vi "Configure Memory Polynomial.vi"(0 "Instrument Handle In":refnum<k21>, 1 "Selector String":string, 5 "Memory Polynomial Configuration":T1={"Correction Type"=0, "Number of Iterations"=3, " Order"=3, " Depth"=2, "Lead Order"=2, "Lag Order"=2, "Lead Memory Depth"=2, "Lag Memory Depth"=2, "Maximum Lead"=2, "Maximum Lag"=2} {"Order" min=1; "Correction Type" items=["Magnitude and Phase", "Magnitude Only", "Phase Only"]}, 11 "error in (no error)":errorcluster) -> (4 "Instrument Handle Out":refnum<k21>, 15 "error out":errorcluster)   [LabVIEW 2016, in "RFmxDPD.lvlib"]
uses:
  RFmxDPD.lvlib
  Typedefs/Memory Polynomial Configuration.ctl
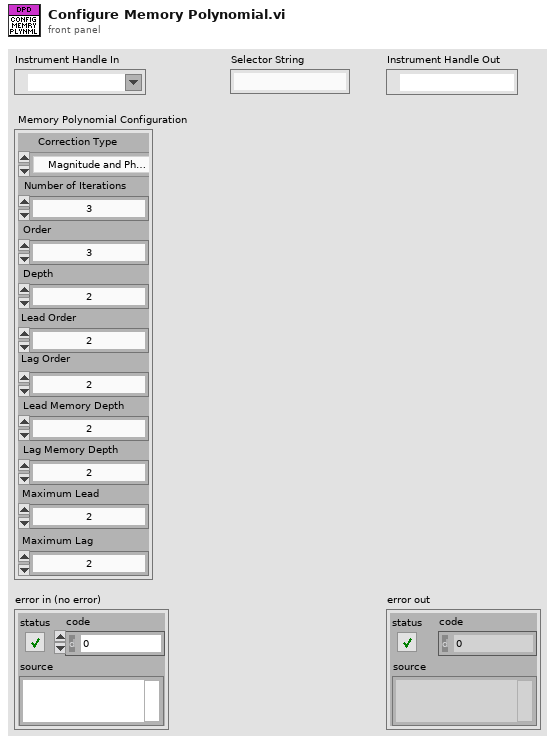
[diagram p1: front panel]
types:
  T1 = typedef "RFmxDPD.lvlib/Memory Polynomial Configuration.ctl" = cluster{"Correction Type":i32, "Number of Iterations":i32, " Order":i32, " Depth":i32, "Lead Order":i32, "Lag Order":i32, "Lead Memory Depth":i32, "Lag Memory Depth":i32, "Maximum Lead":i32, "Maximum Lag":i32}
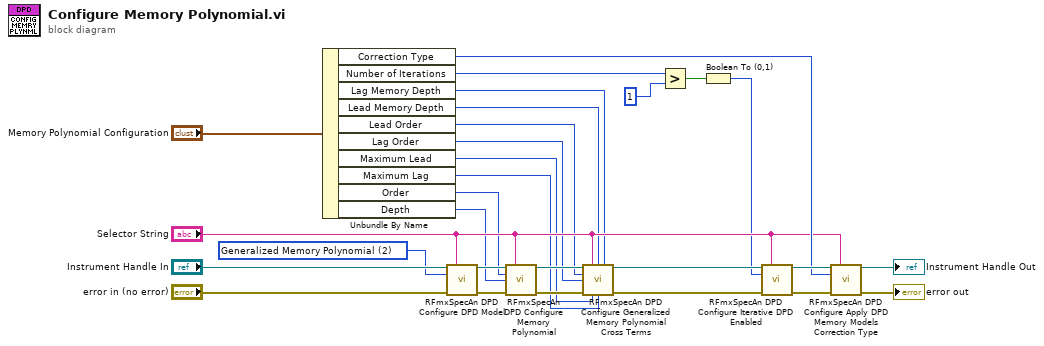
[diagram p0: block diagram]
diagram:
  w18 = 2 items=["Lookup Table", "Memory Polynomial", "Generalized Memory Polynomial"] ("DPD Model")
  n1 = Unbundle By Name("Memory Polynomial Configuration") -> ("Correction Type"=w17:i32, "Number of Iterations"=w4:i32, "Lag Memory Depth"=w15:i32, "Lead Memory Depth"=w14:i32, "Lead Order"=w13:i32, "Lag Order"=w12:i32, "Maximum Lead"=w11:i32, "Maximum Lag"=w10:i32, "Order"=w9:i32, "Depth"=w8:i32)
  n2 = call <vilib>:"RFmxSpecAn DPD Configure DPD Model.vi"("Instrument Handle In"="Instrument Handle In", "Selector String"="Selector String", "DPD Model"=w18, "error in (no error)"="error in (no error)") -> ("Instrument Handle Out"=w25:refnum<k21>, "error out"=w26:errorcluster)  [unwired: 10 in]
  n3 = call <vilib>:"RFmxSpecAn DPD Configure Memory Polynomial.vi"("Instrument Handle In"=w25, "Selector String"="Selector String", "Memory Polynomial Order"=w9, "Memory Polynomial Memory Depth"=w8, "error in (no error)"=w26) -> ("Instrument Handle Out"=w28:refnum<k21>, "error out"=w27:errorcluster)  [unwired: 9 in]
  n4 = call <vilib>:"RFmxSpecAn DPD Configure Generalized Memory Polynomial Cross Terms.vi"("Instrument Handle In"=w28, "Selector String"="Selector String", "Memory Polynomial Lead Memory Depth"=w14, "Memory Polynomial Lag Memory Depth"=w15, "Memory Polynomial Lead Order"=w13, "Memory Polynomial Lag Order"=w12, "error in (no error)"=w27, "Memory Polynomial Max Lead"=w11, "Memory Polynomial Max Lag"=w10) -> ("Instrument Handle Out"=w24:refnum<k21>, "error out"=w23:errorcluster)  [unwired: 5 in]
  n5 = Greater?(x=w4, y=1) -> (0:w2:bool)
  n6 = Boolean To (0,1)(Boolean=w2) -> (0, 1=w1:i16)
  n7 = call <vilib>:"RFmxSpecAn DPD Configure Iterative DPD Enabled.vi"("Instrument Handle In"=w24, "Selector String"="Selector String", "Iterative DPD Enabled"=w1, "error in (no error)"=w23) -> ("Instrument Handle Out"=w22:refnum<k21>, "error out"=w21:errorcluster)  [unwired: 10 in]
  n8 = call <vilib>:"RFmxSpecAn DPD Configure Apply DPD Memory Models Correction Type.vi"("Instrument Handle In"=w22, "Selector String"="Selector String", "Mem Models Correction Type"=w17, "error in (no error)"=w21) -> ("Instrument Handle Out"=→"Instrument Handle Out":refnum<k21>, "error out"=→"error out":errorcluster)  [unwired: 10 in]
